vi "VGA_ganancia.vi"(7 "Espera acceso USB":u32=10, 8 "error in 2":errorcluster, 10 "Ganancia":u8, 11 "ftHandle_in 2":u32) -> (0 "error out 2":errorcluster, 3 "ftHandle_out 2":u32)   [LabVIEW 2019]
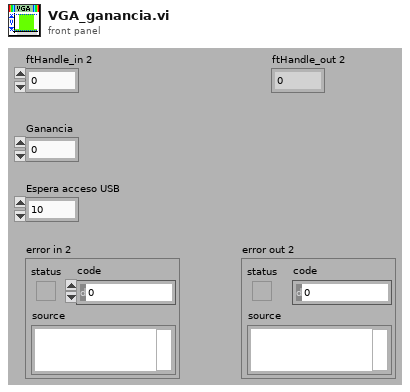
[diagram p1: front panel]
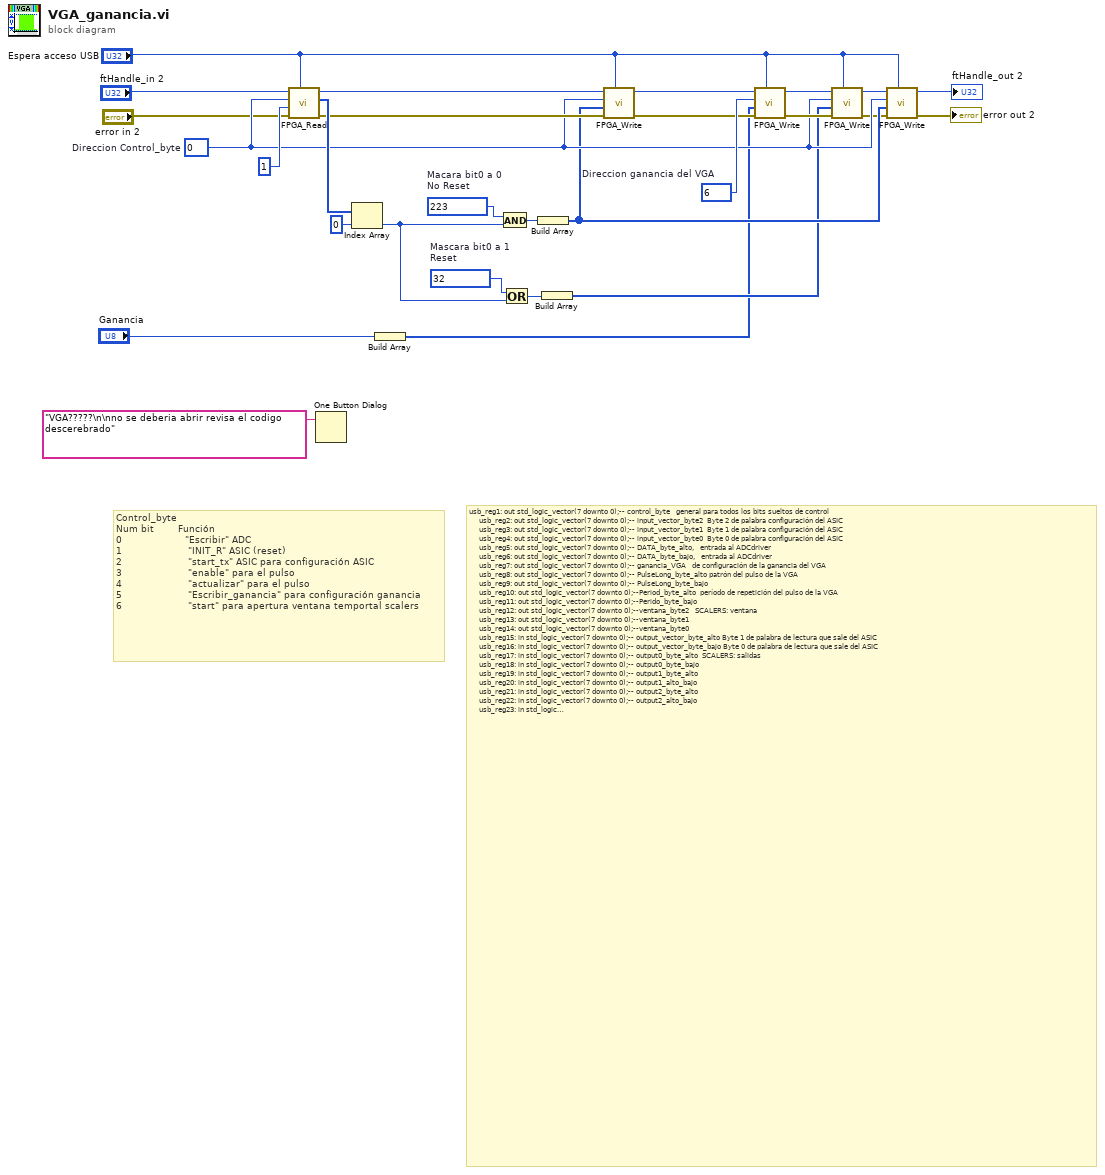
[diagram p0: block diagram]
diagram:
  w28 = u8 6  # Direccion ganancia del VGA
  w23 = u8 32  # Mascara bit0 a 1 Reset
  w21 = u8 223  # Macara bit0 a 0 No Reset
  w13 = u8 0  # Direccion Control_byte
  # "Control_byte\nNum bit        Función\n0                     \"Escribir\" ADC\n1                      \"INIT_R\" ASIC (reset)\n2                      \"start_tx\" ASIC para configuración ASIC\n3                      \"enable\" para el pulso\n4                      \"actualizar\" para el pulso\n5                      \"Escribir_ganancia\" para configuración ganancia\n6                      \"start\" para apertura ventana temportal scalers"
  # "usb_reg1: out std_logic_vector(7 downto 0);-- control_byte\t\t\tgeneral para todos los bits sueltos de control\n\t\t\t  usb_reg2: out std_logic_vector(7 downto 0);-- input_vector_byte2 \tByte 2 de palabra configuración del ASIC\n\t\t\t  usb_reg3: out std_logic_vector(7 downto 0);-- input_vector_byte1 \tByte 1 de palabra configuración del ASIC\n\t\t\t  usb_reg4: out std_logic_vector(7 downto 0);-- input_vector_byte0 \tByte 0 de palabra configuración del ASIC\n\t\t\t  usb_reg5: out std_logic_vector(7 downto 0);-- DATA_byte_alto, \t\tentrada al ADCdriver\n\t\t\t  usb_reg6: out std_logic_vector(7 downto 0);-- DATA_byte_bajo, \t\tentrada al ADCdriver\n\t\t\t  usb_reg7: out std_logic_vector(7 downto 0);-- ganancia_VGA\t\t\tde configuración de la ganancia del VGA\n\t\t\t  usb_reg8: out std_logic_vector(7 downto 0);-- PulseLong_byte_alto\tpatrón del pulso de la VGA\n\t\t\t  usb_reg9: out std_logic_vector(7 downto 0);-- PulseLong_byte_bajo\n\t\t\t  usb_reg10: out std_logic_vector(7 downto 0);--Period_byte_alto\t\tperíodo de repetición del pulso de la VGA\n\t\t\t  usb_reg11: out std_logic_vector(7 downto 0);--Perido_byte_bajo\n\t\t\t  usb_reg12: out std_logic_vector(7 downto 0);--ventana_byte2\t\t\tSCALERS: ventana\n\t\t\t  usb_reg13: out std_logic_vector(7 downto 0);--ventana_byte1\t\n\t\t\t  usb_reg14: out std_logic_vector(7 downto 0);--ventana_byte0\n\t\t\t  usb_reg15: in std_logic_vector(7 downto 0);-- output_vector_byte_alto\tByte 1 de palabra de lectura que sale del ASIC\n\t\t\t  usb_reg16: in std_logic_vector(7 downto 0);-- output_vector_byte_bajo\tByte 0 de palabra de lectura que sale del ASIC\n\t\t\t  usb_reg17: in std_logic_vector(7 downto 0);-- output0_byte_alto\t\tSCALERS: salidas\n\t\t\t  usb_reg18: in std_logic_vector(7 downto 0);-- output0_byte_bajo\n\t\t\t  usb_reg19: in std_logic_vector(7 downto 0);-- output1_byte_alto\n\t\t\t  usb_reg20: in std_logic_vector(7 downto 0);-- output1_alto_bajo \n\t\t\t  usb_reg21: in std_logic_vector(7 downto 0);-- output2_byte_alto \n\t\t\t  usb_reg22: in std_logic_vector(7 downto 0);-- output2_alto_bajo \n\t\t\t  usb_reg23: in std_logic_vector(7 downto 0);-- para el canal_0 del ADCdriver\n\t\t\t  usb_reg24: in std_logic_vector(7 downto 0);\n\t\t\t  usb_reg25: in std_logic_vector(7 downto 0);-- para el canal_1 del ADCdriver\n\t\t\t  usb_reg26: in std_logic_vector(7 downto 0);\n\t\t\t  usb_reg27: in std_logic_vector(7 downto 0);-- para el canal_2 del ADCdriver\n\t\t\t  usb_reg28: in std_logic_vector(7 downto 0);\n\t\t\t  usb_reg29: in std_logic_vector(7 downto 0);-- para el canal_3 del ADCdriver\n\t\t\t  usb_reg30: in std_logic_vector(7 downto 0);\n\t\t\t  usb_reg31: in std_logic_vector(7 downto 0);-- para el canal_4 del ADCdriver\n\t\t\t  usb_reg32: in std_logic_vector(7 downto 0);\n\t\t\t  usb_reg33: in std_logic_vector(7 downto 0);-- para el canal_5 del ADCdriver\n\t\t\t  usb_reg34: in std_logic_vector(7 downto 0);\n\t\t\t  usb_reg35: in std_logic_vector(7 downto 0);-- para el canal_6 del ADCdriver\n\t\t\t  usb_reg36: in std_logic_vector(7 downto 0);\n\t\t\t  usb_reg37: in std_logic_vector(7 downto 0);-- para el canal_7 del ADCdriver\n\t\t\t  usb_reg38: in std_logic_vector(7 downto 0);\n\t\t\t  usb_reg39: in std_logic_vector(7 downto 0);-- para el canal_8 del ADCdriver\n\t\t\t  usb_reg40: in std_logic_vector(7 downto 0);\n\t\t\t  usb_reg41: in std_logic_vector(7 downto 0);-- para el canal_9 del ADCdriver\n\t\t\t  usb_reg42: in std_logic_vector(7 downto 0);\n\t\t\t  usb_reg43: in std_logic_vector(7 downto 0);-- para el canal_10 del ADCdriver\n\t\t\t  usb_reg44: in std_logic_vector(7 downto 0)--;"
  n1 = call "FPGA_Read.vi"("Espera acceso USB"="Espera acceso USB", "error in"="error in 2", "Numero Bytes"=u8 1, "Dirección base"=w13, "ftHandle_in"="ftHandle_in 2") -> ("error out"=w16:errorcluster, "lpBuffer_out"=w17:u8[], "ftHandle_out"=w15:u32)  [unwired: 2 in, 2 out]
  n2 = One Button Dialog(message="VGA?????\n\nno se deberia abrir revisa el codigo descerebrado") -> ()  [unwired: 1 in, 1 out]
  n3 = Index Array(array=w17, index=0) -> (element=w22:u8)
  n4 = Build Array("Ganancia") -> (w3:u8[])
  n5 = And(x=w21, y=w22) -> (x .and. y?=w19:u8)
  n6 = Or(x=w23, y=w22) -> (x .or. y?=w20:u8)
  n7 = Build Array(w19) -> (w12:u8[])
  n8 = Build Array(w20) -> (w9:u8[])
  n9 = call "FPGA_Write.vi"("Espera acceso USB"="Espera acceso USB", "error in"=w16, "Bytes de escritura"=w12, "Dirección base"=w13, "ftHandle_in"=w15) -> ("error out"=w25:errorcluster, "ftHandle_out"=w24:u32)  [unwired: 1 in, 2 out]
  n10 = call "FPGA_Write.vi"("Espera acceso USB"="Espera acceso USB", "error in"=w25, "Bytes de escritura"=w3, "Dirección base"=w28, "ftHandle_in"=w24) -> ("error out"=w27:errorcluster, "ftHandle_out"=w26:u32)  [unwired: 1 in, 2 out]
  n11 = call "FPGA_Write.vi"("Espera acceso USB"="Espera acceso USB", "error in"=w27, "Bytes de escritura"=w9, "Dirección base"=w13, "ftHandle_in"=w26) -> ("error out"=w10:errorcluster, "ftHandle_out"=w11:u32)  [unwired: 1 in, 2 out]
  n12 = call "FPGA_Write.vi"("Espera acceso USB"="Espera acceso USB", "error in"=w10, "Bytes de escritura"=w12, "Dirección base"=w13, "ftHandle_in"=w11) -> ("error out"=→"error out 2":errorcluster, "ftHandle_out"=→"ftHandle_out 2":u32)  [unwired: 1 in, 2 out]
